vi "TP_Init.vi"(8 "error in (no error)":errorcluster, 9 "Constraints":T1, 10 "Unprofiled Goal":T2, 11 "Initial":T2) -> (0 "error out":errorcluster, 3 "TrapezoidalProfile out":refnum<class "TrapezoidalProfile.lvclass">)   [LabVIEW 2018, in "TrapezoidalProfile.lvclass"]
uses:
  TrapezoidalProfile.lvclass
  State.ctl
  Constraints.ctl
  TrapezoidalProfile.lvclass/TrapezoidalProfile.ctl
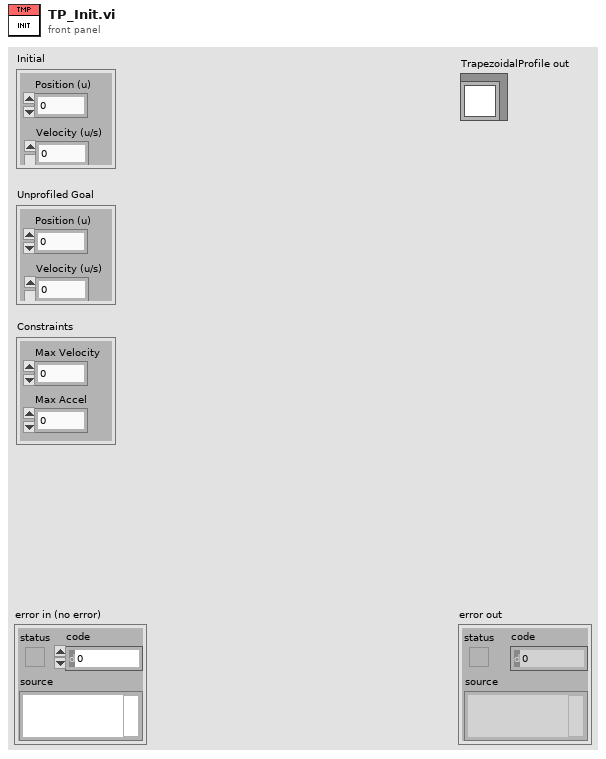
[diagram p1: front panel]
types:
  T1 = typedef "TrapezoidalProfile.lvclass/Constraints.ctl" = cluster{"Max Velocity":dbl, "Max Accel":dbl}
  T2 = typedef "TrapezoidalProfile.lvclass/State.ctl" = cluster{"Position (u)":dbl, "Velocity (u/s)":dbl}
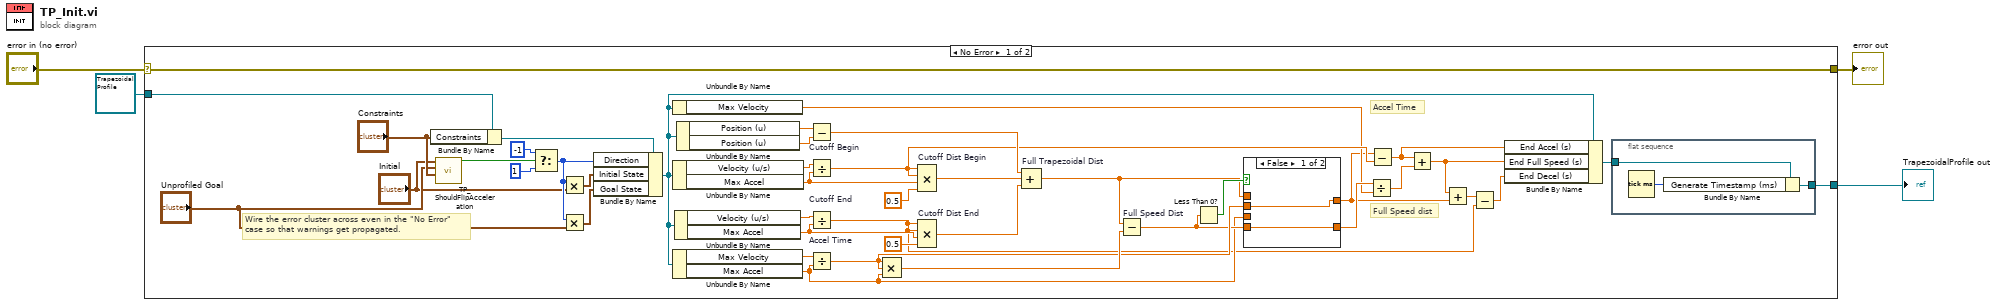
[diagram p0: block diagram]
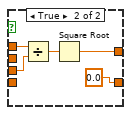
[diagram p2: hidden frame]
diagram:
  n1 = case shown="No Error" "error in (no error)" {
    selector: "error in (no error)" -> [w47 w59]
    tunnel: [w47 w59] -> w3
    tunnel: [w5 w58] -> w1
    tunnel: refnum<class "TrapezoidalProfile.lvclass"> refnum ("OneDimProfile in") -> [w46 w58]
    frame No Error {
      # "Accel Time"
      # "Full Speed dist"
      # "Wire the error cluster across even in the \"No Error\"\ncase so that warnings get propagated."
      n2 = Bundle By Name(cluster=w46, "Constraints"="Constraints") -> (w41:refnum<class "TrapezoidalProfile.lvclass">)
      n3 = call "TP_ShouldFlipAcceleration.vi"("Constraints"="Constraints", "Goal"="Unprofiled Goal", "Initial"="Initial") -> ("Is Accel Flipped?"=w44:bool)  [unwired: 8 in]
      n4 = Select(t=-1, s=w44, f=1) -> (s? t:f=w38:i32)
      n5 = Multiply(x=w38, y="Initial") -> (x*y=w40:T2)
      n6 = Multiply(x=w38, y="Unprofiled Goal") -> (x*y=w39:T2)
      n7 = Bundle By Name(cluster=w41, "Direction"=w38, "Initial State"=w40, "Goal State"=w39) -> (w16:refnum<class "TrapezoidalProfile.lvclass">)
      n8 = Unbundle By Name(w16) -> ("Max Velocity"=w15:dbl)
      n9 = Unbundle By Name(w16) -> ("Velocity (u/s)"=w35:dbl, "Max Accel"=w34:dbl)
      n10 = Unbundle By Name(w16) -> ("Max Velocity"=w25:dbl, "Max Accel"=w19:dbl)
      n11 = Unbundle By Name(w16) -> ("Velocity (u/s)"=w32:dbl, "Max Accel"=w11:dbl)
      n12 = Unbundle By Name(w16) -> ("Position (u)"=w30:dbl, "Position (u)"=w29:dbl)
      n13 = Subtract(x=w30, y=w29) -> (x-y=w28:dbl)
      n14 = Divide "Cutoff Begin"(x=w35, y=w34) -> (x/y=w18:dbl)
      n15 = Divide "Cutoff End"(x=w32, y=w11) -> (x/y=w9:dbl)
      n16 = Divide "Accel Time"(x=w25, y=w19) -> (x/y=w22:dbl)
      n17 = Compound Arithmetic op=MULTIPLY(w22, w22, w19) -> (w24:dbl)
      n18 = Compound Arithmetic op=MULTIPLY "Cutoff Dist Begin"(w18, w18, w34, 0.5 ("value")) -> (w27:dbl)
      n19 = Compound Arithmetic op=MULTIPLY "Cutoff Dist End"(w9, w9, w11, 0.5 ("value")) -> (w26:dbl)
      n20 = Compound Arithmetic op=ADD "Full Trapezoidal Dist"(w28, w27, w26) -> (w20:dbl)
      n21 = Subtract "Full Speed Dist"(x=w20, y=w24) -> (x-y=w21:dbl)
      n22 = Less Than 0?(x=w21) -> (x < 0?=w23:bool)
      n23 = case shown="False" w23 {
        tunnel: w22 -> [w51 _]
        tunnel: w21 -> [w52 _]
        tunnel: [w52 0.0] -> w17
        tunnel: [w51 w56] -> w8
        tunnel: w20 -> [_ w54]
        tunnel: w19 -> [_ w55]
        frame False {
        }
        frame True {
          n24 = Divide(x=w54, y=w55) -> (x/y=w53:dbl)
          n25 = Square Root(x=w53) -> (sqrt(x)=w56:dbl)
        }
      }
      n26 = Divide(x=w17, y=w15) -> (x/y=w13:dbl)
      n27 = Subtract(x=w8, y=w18) -> (x-y=w14:dbl)
      n28 = Add(x=w14, y=w13) -> (x+y=w12:dbl)
      n29 = Add(x=w12, y=w8) -> (x+y=w10:dbl)
      n30 = Subtract(x=w10, y=w9) -> (x-y=w7:dbl)
      n31 = Bundle By Name(cluster=w16, "End Accel (s)"=w14, "End Full Speed (s)"=w12, "End Decel (s)"=w7) -> (w6:refnum<class "TrapezoidalProfile.lvclass">)
      n32 = flat-sequence {
        tunnel: w6 -> [w50]
        tunnel: [w48] -> w5
        frame #0 {
          n33 = Tick Count (ms)() -> (millisecond timer value=w49:u32)
          n34 = Bundle By Name(cluster=w50, "Generate Timestamp (ms)"=w49) -> (w48:refnum<class "TrapezoidalProfile.lvclass">)
        }
      }
    }
    frame Error {
    }
  }
  "error out" <- w3
  "TrapezoidalProfile out" <- w1
